vi "Barcode Scanner.vi"(8 "error in":errorcluster, 10 "DUT":string) -> (0 "error in (out)":errorcluster)   [LabVIEW 2024, in "Barcode_Scanner.lvlib"]
doc: "This template is for the Queued Message Handler design pattern.\n\nThe Event Handling Loop generates messages based on user interface actions.\n\nThe Message Handling Loop processes messages generated by the Event Handling Loop, or by other messages. The messages are string values, so new messages can be added easily to the Message Cases case structure in the Message Handling Loop. Each message cluster can also provide an optional value for Message Data, which is a variant that can be converted to whatever message-specific data is required."
uses:
  Barcode_Scanner.lvlib
  controls/Barcode UI Data.ctl
  <vilib>/Instr/_visa.llb/VISA Flush IO Buffer Mask.ctl
  PrivateControls/FGV_Queue_Control.ctl
  Launcher/SubVI/Global 1.vi
  <vilib>/Instr/_visa.llb/VISA Configure Serial Port (Instr).vi
  <vilib>/Utility/error.llb/Error Cluster From Error Code.vi
  <vilib>/regexp/Match Regular Expression.xnode
  <vilib>/ErrorRing/Error Ring.xnode
  support/Message Queue/Barcode Message Queue.lvlib
  support/User Event - Stop/Barcode User Event - Stop.lvlib
  Launcher/Launcher_DTU.lvlib
panel:
  out "read buffer 2":string
  out "Timer 2":i32
  out "Barcode 2":string
  out "status 2":bool
  out "read buffer":string
  in  "Config":string
  out "status":bool
  out "Barcode":string
  out "Timer":i32
  in  "PLC_name":refnum<visa-resource-name>
  out "queue name 2":string
  out "queue name":string
  out "Display <Replace Me>":string
  in  "DigitalWrite":bool
  in  "Digital Read":bool
  in  "Exit":bool
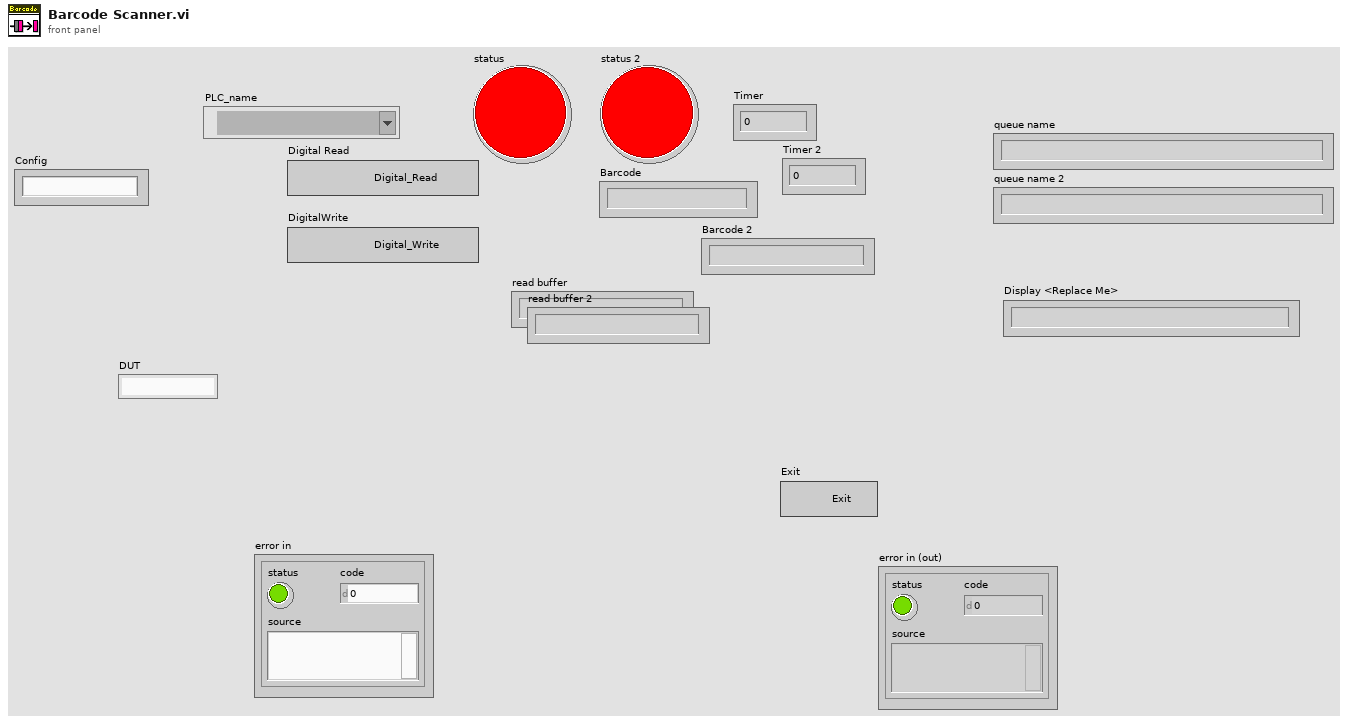
[diagram p1: front panel]
types:
  T1 = typedef "Barcode_Scanner.lvlib/Barcode UI Data.ctl" = cluster{"Config_Path":path, "DUT":i32, "notifier out":refnum<notifier>, "Barcode COM":refnum<visa-resource-name>, "Timer":u32, "queue out":refnum<queue>, "Config":string, "Barcode_path":path, "Barcode_init":bool}
  T2 = typedef "Barcode_Scanner.lvlib/FGV_Queue_Control.ctl" = enum16{"Release", "Get", "Set"}
  T3 = typedef "Barcode_Scanner.lvlib/Barcode Message Queue.lvlib/All Message Queues.ctl" = cluster{"UI":refnum<queue>, "QSM":refnum<queue>}
  T4 = enum16{"Read", "Write", "All_sections", "All_values", "Remove key&section"}
  T5 = cluster{"Message":string, "Message Data":variant}
  T6 = typedef "VISA Flush IO Buffer Mask.ctl" = u16
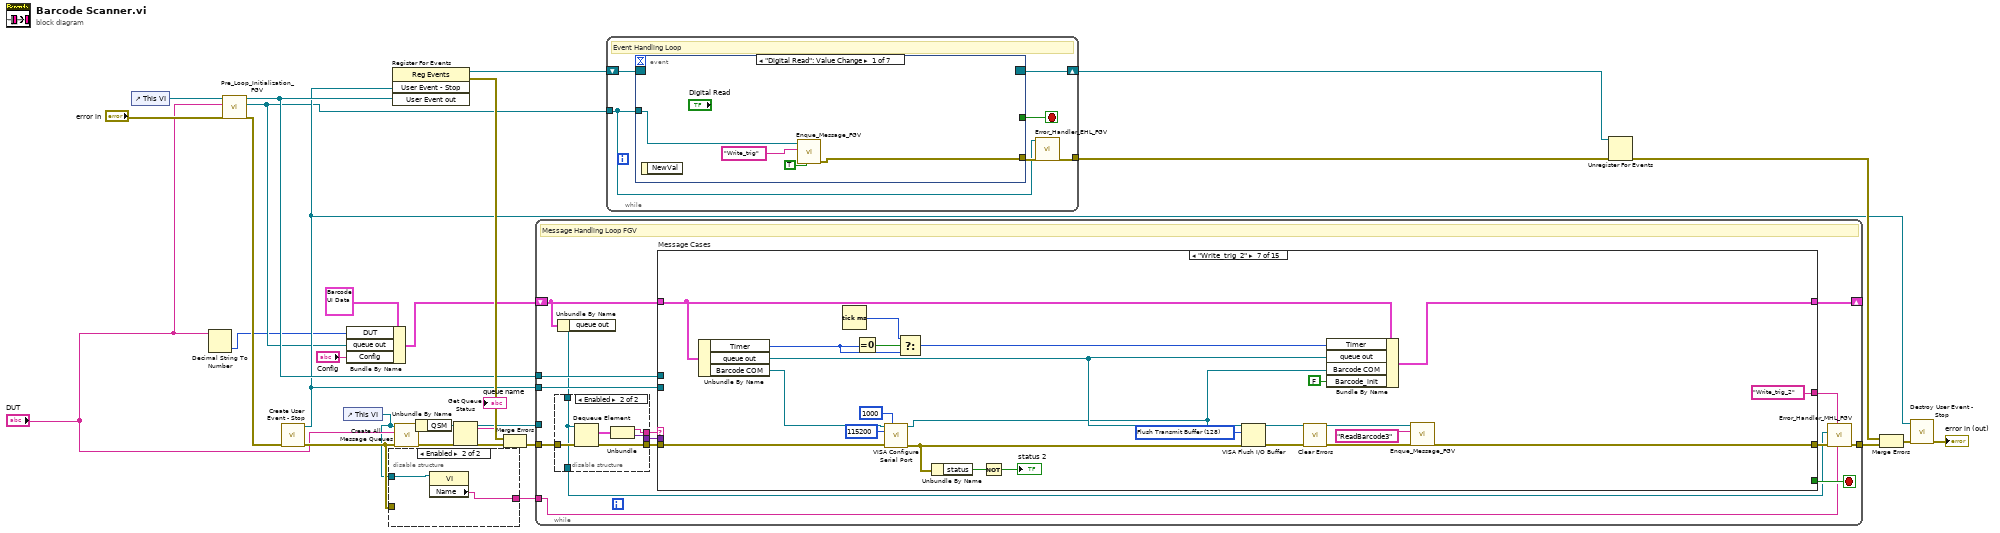
[diagram p0: block diagram]
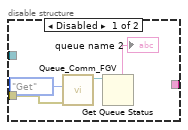
[diagram p2: hidden frame]
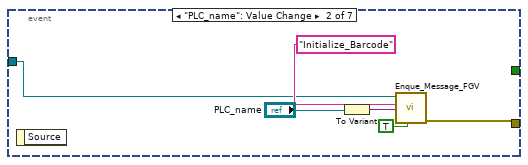
[diagram p3: hidden frame]
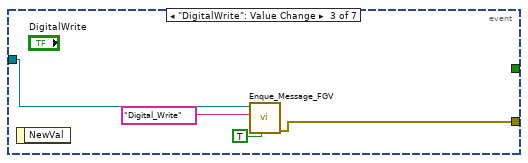
[diagram p4: hidden frame]
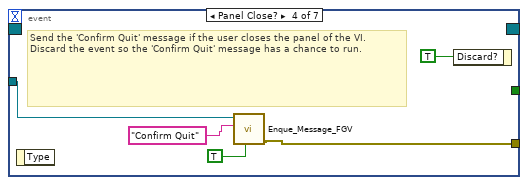
[diagram p5: hidden frame]
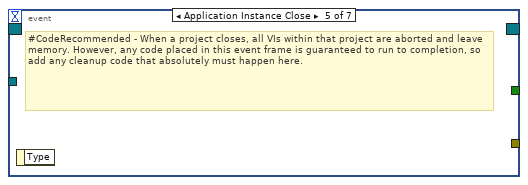
[diagram p6: hidden frame]
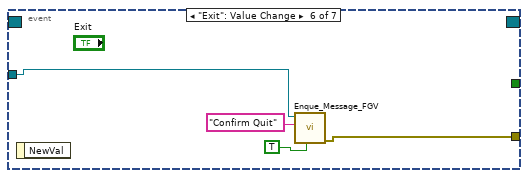
[diagram p7: hidden frame]
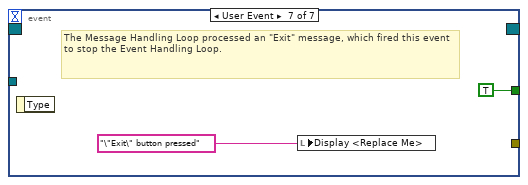
[diagram p8: hidden frame]
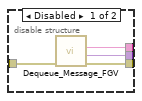
[diagram p9: hidden frame]
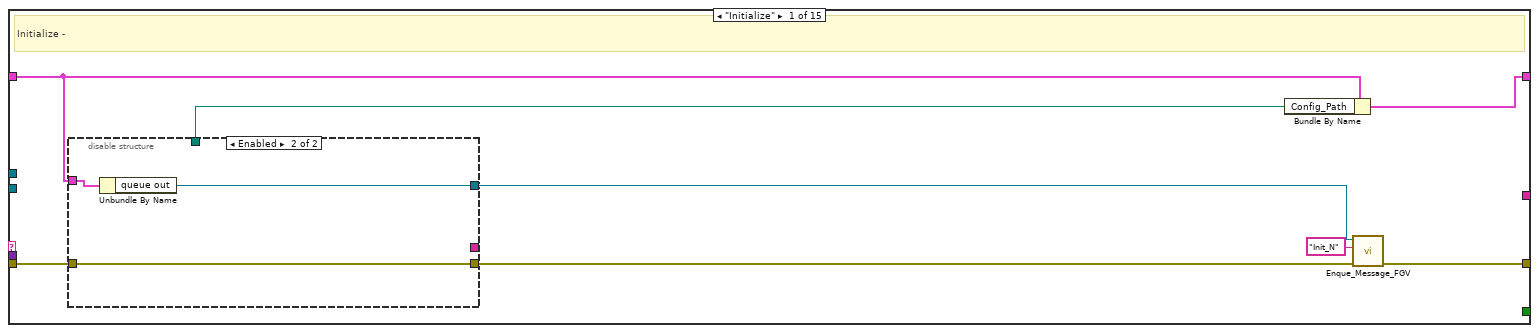
[diagram p10: hidden frame]
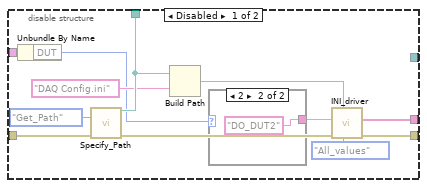
[diagram p11: hidden frame]
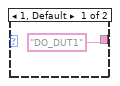
[diagram p12: hidden frame]
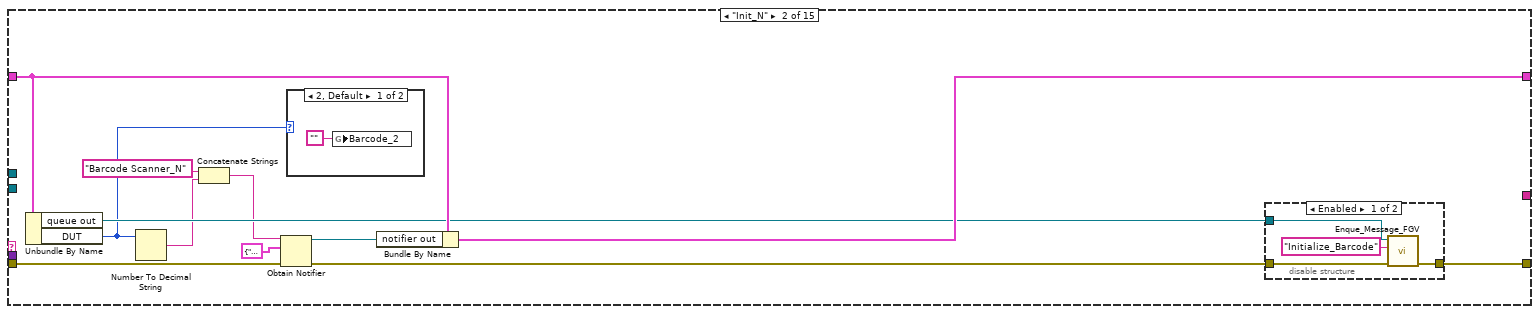
[diagram p13: hidden frame]
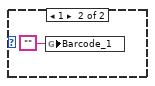
[diagram p14: hidden frame]
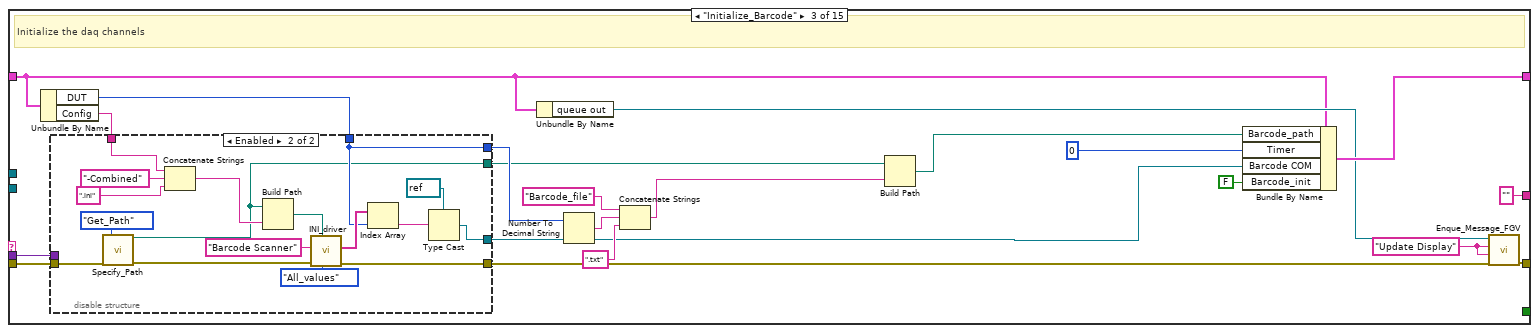
[diagram p16: hidden frame]
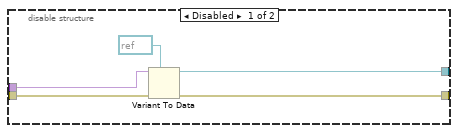
[diagram p17: hidden frame]
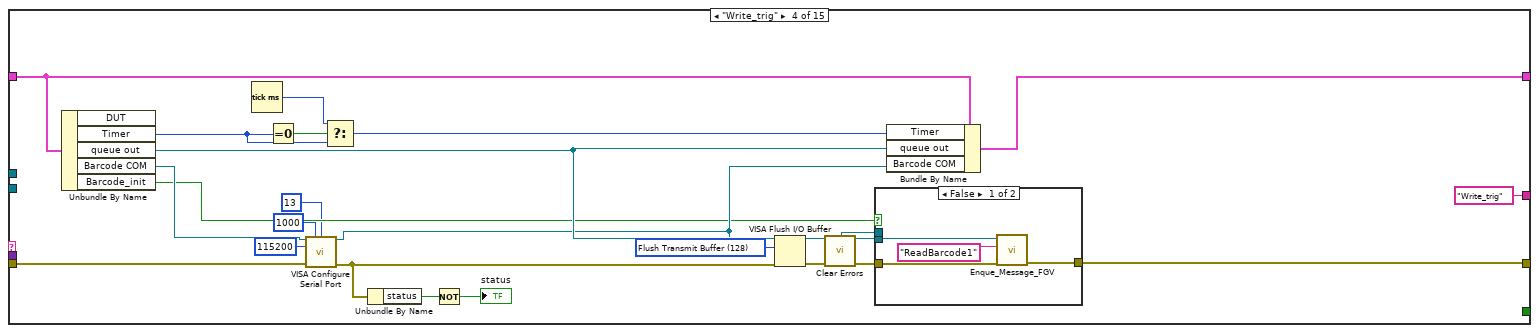
[diagram p18: hidden frame]
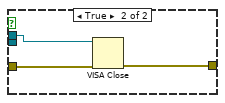
[diagram p19: hidden frame]
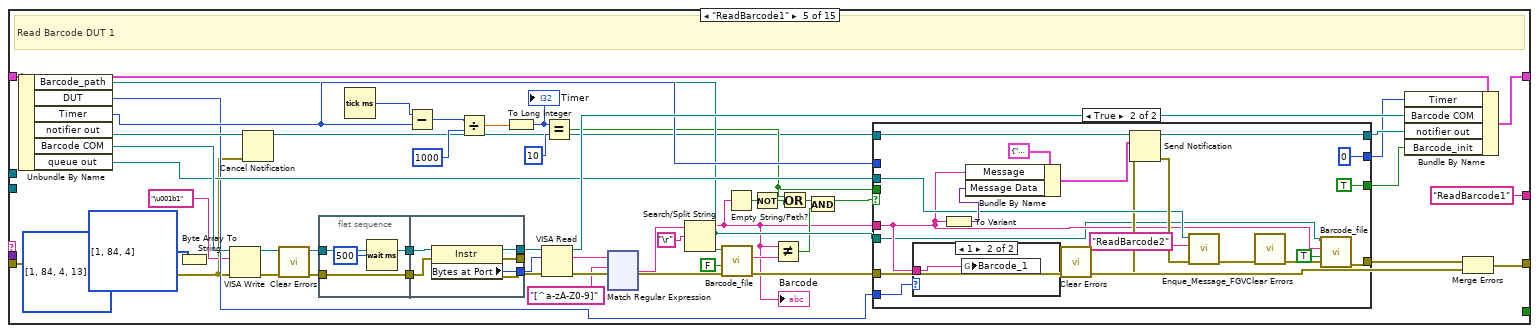
[diagram p20: hidden frame]
diagram:
  n1 = control-ref of="This VI"() -> (w16:refnum<vi>)
  n2 = Decimal String To Number(string="DUT") -> (number=w4:i32)  [unwired: 2 in, 1 out]
  n3 = call "Pre_Loop_Initialization_FGV.vi"("error in (no error)"="error in", "DUT"="DUT", "VI in"=w16) -> ("error out"=w14:errorcluster, "queue out"=w5:refnum<queue>, "User Event out"=w9:refnum<user-event>)  [unwired: 6 in]
  n4 = call "Create User Event - Stop.vi"("error in (no error)"=w14) -> ("error out"=w10:errorcluster, "User Event - Stop"=w8:refnum<user-event>)  [unwired: 9 in]
  n5 = control-ref of="This VI"() -> (w2:refnum<vi>)
  n6 = Bundle By Name(cluster=T1 {"Config_Path"=path "", "DUT"=0, "notifier out"=refnum, "Barcode COM"="", "Timer"=0, "queue out"=refnum, "Config"="", "Barcode_path"=path "", "Barcode_init"=FALSE} ("Data Cluster"), "DUT"=w4, "queue out"=w5, "Config"="Config") -> (w7:T1)
  n7 = disable-structure shown="Enabled" {
    disable-tunnel: w10 -> [w32 _]
    disable-tunnel: w2 -> [_ w34]
    disable-tunnel: [_ w33] -> w1
    frame Disabled {
      n8 = call "Queue_Comm_FGV.vi"("error in (no error)"=w32, "Enum"=FGV_Queue_Control."Get") -> ("queue Out"=w30:refnum<queue>)  [unwired: 8 in, 1 out]
      n9 = Get Queue Status(queue=w30) -> (queue name=→"queue name 2":string)  [unwired: 2 in, 7 out]
    }
    frame Enabled {
      n10 = property class="VI"(reference=w34) -> ("Name"=w33:string)  [unwired: 1 in, 2 out]
    }
  }
  n11 = register-events(w8, w9) -> (reference out=w19:refnum<event-registration>, error out=w17:errorcluster)  [unwired: 2 in]
  n12 = call "Create All Message Queues.vi"("error in (no error)"=w10, "DUT"="DUT", "This VI"=w2) -> ("error out"=w28:errorcluster, "Message Queues out"=w27:T3)  [unwired: 7 in]
  n13 = Unbundle By Name(w27) -> ("QSM"=w25:refnum<queue>)
  n14 = Get Queue Status(queue=w25) -> (queue out=w12:refnum<queue>, queue name=→"queue name":string)  [unwired: 2 in, 6 out]
  n15 = Merge Errors(w17, w28) -> (w18:errorcluster)
  n16 = while {
    tunnel: w12 -> [_]
    shift-right: [w49] -> _
    shift-left: w7 -> [w39]
    tunnel: w9 -> [w47]
    tunnel: w18 -> [w46]
    tunnel: [w41] -> w26
    tunnel: w8 -> [w40]
    tunnel: w1 -> [w35]
    stop <- w48 stop-if-true
    # "Message Handling Loop FGV"
    n17 = Unbundle By Name(w39) -> ("queue out"=w38:refnum<queue>)
    n18 = disable-structure shown="Enabled" {
      disable-tunnel: w46 -> [w53 w59]
      disable-tunnel: [w52 w58] -> w45
      disable-tunnel: [w51 w55] -> w44
      disable-tunnel: [w50 w56] -> w43
      disable-tunnel: w38 -> [_ w54]
      disable-tunnel: [_ w54] -> w37
      frame Disabled {
        n19 = call "Dequeue_Message_FGV.vi"("error in (no error)"=w53) -> ("error out"=w52:errorcluster, "Message Data"=w51:variant, "Message"=w50:string)  [unwired: 8 in]
      }
      frame Enabled {
        n20 = Dequeue Element(queue=w54, error in (no error)=w59) -> (element=w57:T5, error out=w58:errorcluster)  [unwired: 1 in, 2 out]
        n21 = Unbundle(w57) -> ("Message"=w56:string, "Message Data"=w55:variant)
      }
    }
    n22 = case "Message Cases" shown="\"Write_trig_2\"" w43 {
      selector: w43 -> [_ _ _ _ _ _ _ _ _ _ _ _ _ _ w691]
      tunnel: w45 -> [w66 w96 w122 w157 w177 w397 w416 w461 w634 w650 w657 w667 w672 w681 _]
      tunnel: [w67 w90 w124 w163 w222 w402 w422 w469 w639 w651 w657 w661 w674 w678 w692] -> w42
      tunnel: w39 -> [w61 w95 w117 w169 w224 w401 w429 w471 w638 w652 w656 w666 w669 w682 w693]
      tunnel: [w64 w93 w120 w165 w223 w400 w425 w470 w637 w652 w654 w666 w669 w682 w693] -> w49
      tunnel: [_ _ _ _ _ _ _ _ _ _ _ _ _ TRUE _] -> w48
      tunnel: w44 -> [_ _ w121 _ _ _ _ _ _ w649 _ w665 _ _ _]
      tunnel: w47 -> [_ _ _ _ _ _ _ _ _ _ _ _ _ w688 _]
      tunnel: w40 -> [_ _ _ _ _ _ _ _ _ _ _ _ _ w685 _]
      tunnel: [_ _ "" "Write_trig" "ReadBarcode1" "ReadBarcode2" "Write_trig_2" "ReadBarcode3" "ReadBarcode4" "" _ _ _ _ _] -> w36
      frame "Initialize" {
        # "Initialize -"
        n23 = disable-structure shown="Enabled" {
          disable-tunnel: w66 -> [w79 w84]
          disable-tunnel: [w76 w84] -> w63
          disable-tunnel: [w75 _] -> w62
          disable-tunnel: w61 -> [w71 w83]
          disable-tunnel: [w69 _] -> _
          disable-tunnel: [_ w82] -> w60
          frame Disabled {
            n24 = Unbundle By Name(w71) -> ("DUT"=w68:i32)
            n25 = call "Specify_Path.vi"("Path_Enum"=enum16{"Find_Path", "Get_Path"}."Get_Path", "error in (no error)"=w79) -> ("Configurations"=w75:path, "error out"=w78:errorcluster)  [unwired: 6 in, 6 out]
            n26 = Build Path(base path=w75, name or relative path="DAQ Config.ini") -> (appended path=w73:path)
            n27 = case shown="2" w68 {
              tunnel: ["DO_DUT1" ("String") "DO_DUT2" ("String")] -> w70
              frame 1, Default {
              }
              frame 2 {
              }
            }
            n28 = call "INI_driver.vi"("Enum"=T4."All_values", "instrument file path"=w73, "error in (no error)"=w78, "Section"=w70) -> ("error out"=w76:errorcluster, "Values out"=w69:string[])  [unwired: 4 in, 2 out]
          }
          frame Enabled {
            n29 = Unbundle By Name(w83) -> ("queue out"=w82:refnum<queue>)
          }
        }
        n30 = Bundle By Name(cluster=w61, "Config_Path"=w62) -> (w64:T1)
        n31 = call "Enque_Message_FGV.vi"("error in (no error)"=w63, "Message"="Init_N", "queue Out"=w60) -> ("error out"=w67:errorcluster)  [unwired: 8 in]
      }
      frame "Init_N" {
        n32 = Unbundle By Name(w95) -> ("queue out"=w88:refnum<queue>, "DUT"=w85:i32)
        n33 = Number To Decimal String(number=w85) -> (decimal integer string=w86:string)  [unwired: 1 in]
        n34 = Concatenate Strings("Barcode Scanner_N" ("String"), w86) -> (w87:string)
        n35 = Obtain Notifier(name (unnamed)=w87, notification data type=T5 {"Message"="", "Message Data"=variant} ("notification"), error in (no error)=w96) -> (notifier out=w92:refnum<notifier>, error out=w91:errorcluster)  [unwired: 1 in, 1 out]
        n36 = case shown="2, Default" w85 {
          frame 2, Default {
            n37 = global write "Global 1.vi" "Barcode_2"("") -> ()
          }
          frame 1 {
            n38 = global write "Global 1.vi" "Barcode_1"("") -> ()
          }
        }
        n39 = Bundle By Name(cluster=w95, "notifier out"=w92) -> (w93:T1)
        n40 = disable-structure shown="Enabled" {
          disable-tunnel: w91 -> [w101 w103]
          disable-tunnel: [w100 w103] -> w90
          disable-tunnel: w88 -> [w99 _]
          frame Enabled {
            n41 = call "Enque_Message_FGV.vi"("error in (no error)"=w101, "Message"="Initialize_Barcode", "queue Out"=w99) -> ("error out"=w100:errorcluster)  [unwired: 8 in]
          }
          frame Disabled {
          }
        }
      }
      frame "Initialize_Barcode" {
        w123 = "Update Display" ("Message")
        # "Initialize the daq channels"
        n42 = Unbundle By Name(w117) -> ("DUT"=w115:i32, "Config"=w116:string)
        n43 = disable-structure shown="Enabled" {
          disable-tunnel: w122 -> [w129 w136]
          disable-tunnel: [w128 w135] -> w106
          disable-tunnel: w121 -> [w127 _]
          disable-tunnel: [w125 w134] -> w107
          disable-tunnel: w116 -> [_ w133]
          disable-tunnel: w115 -> [_ w131]
          disable-tunnel: [_ w131] -> w114
          disable-tunnel: [_ w130] -> w109
          frame Disabled {
            n44 = Variant To Data(error in=w129, type=refnum<visa-resource-name> refnum ("PLC_name"), Variant=w127) -> (data=w125:refnum<visa-resource-name>, error out=w128:errorcluster)
          }
          frame Enabled {
            n45 = call "Specify_Path.vi"("Path_Enum"=enum16{"Find_Path", "Get_Path"}."Get_Path", "error in (no error)"=w136) -> ("Configurations"=w130:path, "error out"=w143:errorcluster)  [unwired: 6 in, 6 out]
            n46 = Concatenate Strings(w133, "-Combined", ".ini" ("string")) -> (w137:string)
            n47 = Build Path(base path=w130, name or relative path=w137) -> (appended path=w145:path)
            n48 = call "INI_driver.vi"("Enum"=T4."All_values", "instrument file path"=w145, "error in (no error)"=w143, "Section"="Barcode Scanner") -> ("error out"=w135:errorcluster, "Values out"=w141:string[])  [unwired: 4 in, 2 out]
            n49 = Index Array(array=w141, index=w131) -> (element=w140:string)
            n50 = Type Cast(type=refnum<visa-resource-name> refnum ("VISA resource name"), x=w140) -> (*(type *) &x=w134:refnum<visa-resource-name>)
          }
        }
        n51 = Unbundle By Name(w117) -> ("queue out"=w118:refnum<queue>)
        n52 = Number To Decimal String(number=w114) -> (decimal integer string=w111:string)  [unwired: 1 in]
        n53 = Concatenate Strings("Barcode_file", w111, ".txt" ("string")) -> (w113:string)
        n54 = Build Path(base path=w109, name or relative path=w113) -> (appended path=w108:path)
        n55 = Bundle By Name(cluster=w117, "Barcode_path"=w108, "Timer"=u32 0, "Barcode COM"=w107, "Barcode_init"=FALSE) -> (w120:T1)
        n56 = call "Enque_Message_FGV.vi"("error in (no error)"=w106, "Message Data"=w123, "Message"=w123, "queue Out"=w118) -> ("error out"=w124:errorcluster)  [unwired: 7 in]
      }
      frame "Write_trig" {
        w160 = T6 128 items=["Flush Receive Buffer"=16, "Write Transmit Buffer to Device"=32, "Flush Receive Buffer (No I/O)"=64, "Flush Transmit Buffer"=128] ("Mask")
        n57 = Unbundle By Name(w169) -> ("Timer"=w166:u32, "queue out"=w162:refnum<queue>, "Barcode COM"=w156:refnum<visa-resource-name>, "Barcode_init"=w151:bool)  [unwired: 1 out]
        n58 = Tick Count (ms)() -> (millisecond timer value=w167:u32)
        n59 = Equal To 0?(x=w166) -> (x = 0?=w168:bool)
        n60 = call-poly "VISA Configure Serial Port"("VISA resource name"=w156, "timeout (10sec)"=u32 1000, "termination char\n(0xA = '\\n' = LF)"=u8 13 ("termination char\n(0xA = '\\n' = LF)"), "baud rate (9600)"=u32 115200, "error in (no error)"=w157) -> ("VISA resource name out"=w155:refnum<visa-resource-name>, "error out"=w152:errorcluster)  [unwired: 9 in]
        n61 = Select(t=w167, s=w168, f=w166) -> (s? t:f=w164:u32)
        n62 = Unbundle By Name(w152) -> ("status"=w154:bool)
        n63 = Not(x=w154) -> (.not. x?=→"status":bool)
        n64 = VISA Flush I/O Buffer(VISA resource name=w155, mask (16)=w160, error in (no error)=w152) -> (VISA resource name out=w150:refnum<visa-resource-name>, error out=w161:errorcluster)
        n65 = call <vilib>:"Clear Errors.vi"("error in (no error)"=w161) -> ("error out"=w147:errorcluster)  [unwired: 5 in, 1 out]
        n66 = case shown="False" w151 {
          tunnel: [w172 w175] -> w163
          tunnel: w162 -> [w171 _]
          tunnel: w147 -> [w170 w176]
          tunnel: w150 -> [_ w174]
          frame False {
            n67 = call "Enque_Message_FGV.vi"("error in (no error)"=w170, "Message"="ReadBarcode1", "queue Out"=w171) -> ("error out"=w172:errorcluster)  [unwired: 8 in]
          }
          frame True {
            n68 = VISA Close(VISA resource name=w174, error in (no error)=w176) -> (error out=w175:errorcluster)
          }
        }
        n69 = Bundle By Name(cluster=w169, "Timer"=w164, "queue out"=w162, "Barcode COM"=w155) -> (w165:T1)
      }
      frame "ReadBarcode1" {
        (unwired) u8[] [1, 84, 4, 13] ("unsigned byte array")
        # "Read Barcode DUT 1"
        n70 = Unbundle By Name(w224) -> ("Barcode_path"=w191:path, "DUT"=w194:i32, "Timer"=w197:u32, "notifier out"=w221:refnum<notifier>, "Barcode COM"=w214:refnum<visa-resource-name>, "queue out"=w198:refnum<queue>)
        n71 = Byte Array To String(unsigned byte array=u8[] [1, 84, 4]) -> ()  [unwired: 1 out]
        n72 = VISA Write(VISA resource name=w214, write buffer="\u001b1", error in (no error)=w177) -> (VISA resource name out=w213:refnum<visa-resource-name>, error out=w212:errorcluster)  [unwired: 1 out]
        n73 = Cancel Notification(0:w221, 3:w177) -> (8:w178:refnum<notifier>)  [unwired: 2 out]
        n74 = call <vilib>:"Clear Errors.vi"("error in (no error)"=w212) -> ("error out"=w208:errorcluster)  [unwired: 5 in, 1 out]
        n75 = flat-sequence {
          tunnel: w208 -> [w374]
          tunnel: w213 -> [w375]
          tunnel: [w375] -> w210
          tunnel: [w374] -> w209
          tunnel: [w380] -> w218
          tunnel: [w379] -> w217
          tunnel: [w378] -> w216
          tunnel: w210 -> [w377]
          tunnel: w209 -> [w376]
          frame #0 {
            n76 = Wait (ms)(milliseconds to wait=u32 500) -> ()  [unwired: 1 out]
          }
          frame #1 {
            n77 = property class="Instr"(reference=w377, error in=w376) -> (reference out=w380:refnum<visa-resource-name>, error out=w378:errorcluster, "Bytes at Port"=w379:u32)
          }
        }
        n78 = Tick Count (ms)() -> (millisecond timer value=w204:u32)
        n79 = Subtract(x=w204, y=w197) -> (x-y=w203:u32)
        n80 = Divide(x=w203, y=u32 1000) -> (x/y=w201:dbl)
        n81 = To Long Integer(number=w201) -> (32bit integer=w200:i32)
        "Timer" <- w200
        n82 = VISA Read(VISA resource name=w218, byte count=w217, error in (no error)=w216) -> (VISA resource name out=w215:refnum<visa-resource-name>, read buffer=w182:string, error out=w193:errorcluster)  [unwired: 1 out]
        n83 = Equal?(x=w200, y=10) -> (x = y?=w188:bool)
        n84 = xnode "Match Regular Expression"("input string"=w182, "regular expression"="[^a-zA-Z0-9]") -> ("after match"=w181:string)  [unwired: 4 in, 4 out]
        n85 = Search/Split String(string=w181, search string/char (-)="\r") -> (substring before match=w180:string)  [unwired: 1 in, 2 out]
        "Barcode" <- w180
        n86 = call "Barcode_file.vi"("error in"=w193, "Read/Write(Read(F))"=FALSE, "Barcode_Path"=w191) -> ("error out"=w192:errorcluster, "Read_Barcode"=w186:string)  [unwired: 7 in]
        n87 = Empty String/Path?(string/path=w180) -> (empty?=w207:bool)
        n88 = Not(x=w207) -> (.not. x?=w205:bool)
        n89 = Not Equal?(x=w180, y=w186) -> (x != y?=w189:bool)
        n90 = Or(x=w188, y=w205) -> (x .or. y?=w206:bool)
        n91 = And(x=w206, y=w189) -> (x .and. y?=w190:bool)
        n92 = case shown="True" w190 {
          tunnel: w178 -> [w351 w370]
          tunnel: [w349 w353] -> w220
          tunnel: [w351 w367] -> w219
          tunnel: w192 -> [w350 w358]
          tunnel: w180 -> [_ w356]
          tunnel: w198 -> [w348 w362]
          tunnel: w197 -> [w347 _]
          tunnel: [w347 u32 0 ("Timer")] -> w196
          tunnel: w194 -> [_ w361]
          tunnel: w191 -> [_ w355]
          tunnel: w188 -> [w343 _]
          tunnel: [FALSE ("Barcode_init") TRUE ("Barcode_init")] -> w185
          frame False {
            n93 = Select(t="ReadBarcode2" ("Message"), s=w343, f="Write_trig" ("Message")) -> (s? t:f=w344:string)
            n94 = call "Enque_Message_FGV.vi"("error in (no error)"=w350, "Message"=w344, "queue Out"=w348) -> ("error out"=w349:errorcluster)  [unwired: 8 in]
          }
          frame True {
            n95 = case shown="1" w361 {
              tunnel: w356 -> [w371 w372]
              frame 2, Default {
                n96 = global write "Global 1.vi" "Barcode_2"(w371) -> ()
              }
              frame 1 {
                n97 = global write "Global 1.vi" "Barcode_1"(w372) -> ()
              }
            }
            n98 = To Variant(anything=w356) -> (Variant=w366:variant)
            n99 = Bundle By Name(cluster=T5 {"Message"="", "Message Data"=variant} ("notification"), "Message"=w356, "Message Data"=w366) -> (w368:T5)
            n100 = call <vilib>:"Clear Errors.vi"("error in (no error)"=w358) -> ("error out"=w360:errorcluster)  [unwired: 5 in, 1 out]
            n101 = Send Notification(notification=w368, notifier=w370, error in (no error)=w360) -> (notifier out=w367:refnum<notifier>, error out=w363:errorcluster)
            n102 = call "Enque_Message_FGV.vi"("error in (no error)"=w363, "Message"="ReadBarcode2", "queue Out"=w362) -> ("error out"=w354:errorcluster)  [unwired: 8 in]
            n103 = call <vilib>:"Clear Errors.vi"("error in (no error)"=w354) -> ("error out"=w352:errorcluster)  [unwired: 5 in, 1 out]
            n104 = call "Barcode_file.vi"("error in"=w352, "Read/Write(Read(F))"=TRUE, "Barcode"=w356, "Barcode_Path"=w355) -> ("error out"=w353:errorcluster)  [unwired: 6 in, 1 out]
          }
        }
        n105 = Bundle By Name(cluster=w224, "Timer"=w196, "Barcode COM"=w215, "notifier out"=w219, "Barcode_init"=w185) -> (w223:T1)
        n106 = Merge Errors(w220, w192) -> (w222:errorcluster)
      }
      frame "ReadBarcode2" {
        w390 = T6 128 items=["Flush Receive Buffer"=16, "Write Transmit Buffer to Device"=32, "Flush Receive Buffer (No I/O)"=64, "Flush Transmit Buffer"=128] ("Mask")
        # "Read Barcode DUT 2"
        n107 = Unbundle By Name(w401) -> ("notifier out"=w398:refnum<notifier>, "Barcode COM"=w388:refnum<visa-resource-name>, "queue out"=w385:refnum<queue>)
        n108 = property class="Instr"(reference=w388, error in=w397) -> (reference out=w396:refnum<visa-resource-name>, error out=w394:errorcluster, "Bytes at Port"=w395:u32)
        n109 = VISA Read(VISA resource name=w396, byte count=w395, error in (no error)=w394) -> (VISA resource name out=w392:refnum<visa-resource-name>, read buffer=→"read buffer":string, error out=w393:errorcluster)  [unwired: 1 out]
        n110 = VISA Flush I/O Buffer(VISA resource name=w392, mask (16)=w390, error in (no error)=w393) -> (VISA resource name out=w387:refnum<visa-resource-name>, error out=w389:errorcluster)
        n111 = VISA Close(VISA resource name=w387, error in (no error)=w389) -> (error out=w381:errorcluster)
        n112 = Cancel Notification(0:w398, 3:w381) -> (8:w382:refnum<notifier>)  [unwired: 2 out]
        n113 = Flush Queue(queue=w385, error in (no error)=w381) -> (error out=w386:errorcluster)  [unwired: 2 out]
        n114 = Merge Errors(w386, w386) -> (w399:errorcluster)
        n115 = Bundle By Name(cluster=w401, "Barcode COM"=w387, "notifier out"=w382, "Barcode_init"=FALSE) -> (w400:T1)
        n116 = disable-structure shown="Enabled" {
          disable-tunnel: [w406 w407] -> w402
          disable-tunnel: w399 -> [w403 w407]
          frame Disabled {
            n117 = call "Enque_Message_FGV.vi"("error in (no error)"=w403, "Message Data"="Digital_Write1" ("\"Do Something Else\" button pressed"), "Message"="Data_Read") -> ("error out"=w406:errorcluster)  [unwired: 8 in]
          }
          frame Enabled {
          }
        }
      }
      frame "Write_trig_2" {
        w419 = T6 128 items=["Flush Receive Buffer"=16, "Write Transmit Buffer to Device"=32, "Flush Receive Buffer (No I/O)"=64, "Flush Transmit Buffer"=128] ("Mask")
        n118 = Unbundle By Name(w429) -> ("Timer"=w426:u32, "queue out"=w421:refnum<queue>, "Barcode COM"=w415:refnum<visa-resource-name>)
        n119 = Tick Count (ms)() -> (millisecond timer value=w427:u32)
        n120 = Equal To 0?(x=w426) -> (x = 0?=w428:bool)
        n121 = call-poly "VISA Configure Serial Port"("VISA resource name"=w415, "timeout (10sec)"=u32 1000, "baud rate (9600)"=u32 115200, "error in (no error)"=w416) -> ("VISA resource name out"=w414:refnum<visa-resource-name>, "error out"=w411:errorcluster)  [unwired: 10 in]
        n122 = Select(t=w427, s=w428, f=w426) -> (s? t:f=w424:u32)
        n123 = Unbundle By Name(w411) -> ("status"=w413:bool)
        n124 = Not(x=w413) -> (.not. x?=→"status 2":bool)
        n125 = VISA Flush I/O Buffer(VISA resource name=w414, mask (16)=w419, error in (no error)=w411) -> (error out=w420:errorcluster)  [unwired: 1 out]
        n126 = call <vilib>:"Clear Errors.vi"("error in (no error)"=w420) -> ("error out"=w408:errorcluster)  [unwired: 5 in, 1 out]
        n127 = Bundle By Name(cluster=w429, "Timer"=w424, "queue out"=w421, "Barcode COM"=w414, "Barcode_init"=FALSE) -> (w425:T1)
        n128 = call "Enque_Message_FGV.vi"("error in (no error)"=w408, "Message"="ReadBarcode3", "queue Out"=w421) -> ("error out"=w422:errorcluster)  [unwired: 8 in]
      }
      frame "ReadBarcode3" {
        # "Read Barcode DUT 1"
        n129 = Unbundle By Name(w471) -> ("Barcode_path"=w439:path, "DUT"=w440:i32, "Timer"=w443:u32, "notifier out"=w468:refnum<notifier>, "Barcode COM"=w460:refnum<visa-resource-name>, "queue out"=w444:refnum<queue>)  [unwired: 1 out]
        n130 = Byte Array To String(unsigned byte array=u8[] [1, 84, 4, 13]) -> ()  [unwired: 1 out]
        n131 = VISA Write(VISA resource name=w460, write buffer="\u001b1", error in (no error)=w461) -> (VISA resource name out=w459:refnum<visa-resource-name>, error out=w458:errorcluster)  [unwired: 1 out]
        n132 = Cancel Notification(0:w468) -> (8:w430:refnum<notifier>)  [unwired: 1 in, 2 out]
        n133 = call <vilib>:"Clear Errors.vi"("error in (no error)"=w458) -> ("error out"=w454:errorcluster)  [unwired: 5 in, 1 out]
        n134 = flat-sequence {
          tunnel: w454 -> [w615]
          tunnel: w459 -> [w616]
          tunnel: [w616] -> w456
          tunnel: [w615] -> w455
          tunnel: [w621] -> w465
          tunnel: [w620] -> w464
          tunnel: [w619] -> w463
          tunnel: w456 -> [w618]
          tunnel: w455 -> [w617]
          frame #0 {
            n135 = Wait (ms)(milliseconds to wait=u32 500) -> ()  [unwired: 1 out]
          }
          frame #1 {
            n136 = property class="Instr"(reference=w618, error in=w617) -> (reference out=w621:refnum<visa-resource-name>, error out=w619:errorcluster, "Bytes at Port"=w620:u32)
          }
        }
        n137 = Tick Count (ms)() -> (millisecond timer value=w450:u32)
        n138 = Subtract(x=w450, y=w443) -> (x-y=w449:u32)
        n139 = Divide(x=w449, y=u32 1000) -> (x/y=w447:dbl)
        n140 = To Long Integer(number=w447) -> (32bit integer=w446:i32)
        "Timer 2" <- w446
        n141 = VISA Read(VISA resource name=w465, byte count=w464, error in (no error)=w463) -> (VISA resource name out=w462:refnum<visa-resource-name>, read buffer=w435:string, error out=w437:errorcluster)  [unwired: 1 out]
        n142 = Equal?(x=w446, y=10) -> (x = y?=w438:bool)
        n143 = xnode "Match Regular Expression"("input string"=w435, "regular expression"="[^a-zA-Z0-9]") -> ("after match"=w434:string)  [unwired: 4 in, 4 out]
        n144 = Empty String/Path?(string/path=w434) -> (empty?=w453:bool)
        n145 = Not(x=w453) -> (.not. x?=w451:bool)
        n146 = Search/Split String(string=w434, search string/char (-)="\r") -> (substring before match=w432:string)  [unwired: 1 in, 2 out]
        "Barcode 2" <- w432
        n147 = Or(x=w438, y=w451) -> (x .or. y?=w452:bool)
        n148 = case shown="True" w452 {
          tunnel: w430 -> [w597 w611]
          tunnel: [w595 w603] -> w467
          tunnel: [w597 w608] -> w466
          tunnel: w437 -> [w596 w598]
          tunnel: w432 -> [_ w599]
          tunnel: w444 -> [w594 w602]
          tunnel: w443 -> [w593 _]
          tunnel: [w593 u32 0 ("Timer")] -> w442
          tunnel: w440 -> [_ w601]
          tunnel: w439 -> [_ _]
          tunnel: w438 -> [w589 _]
          frame False {
            n149 = Select(t="ReadBarcode4" ("Message"), s=w589, f="Write_trig_2" ("Message")) -> (s? t:f=w590:string)
            n150 = call "Enque_Message_FGV.vi"("error in (no error)"=w596, "Message"=w590, "queue Out"=w594) -> ("error out"=w595:errorcluster)  [unwired: 8 in]
          }
          frame True {
            n151 = case shown="1" w601 {
              tunnel: w599 -> [w612 w613]
              frame 2, Default {
                n152 = global write "Global 1.vi" "Barcode_2"(w612) -> ()
              }
              frame 1 {
                n153 = global write "Global 1.vi" "Barcode_1"(w613) -> ()
              }
            }
            n154 = To Variant(anything=w599) -> (Variant=w607:variant)
            n155 = Bundle By Name(cluster=T5 {"Message"="", "Message Data"=variant} ("notification"), "Message"=w599, "Message Data"=w607) -> (w609:T5)
            n156 = call <vilib>:"Clear Errors.vi"("error in (no error)"=w598) -> ("error out"=w600:errorcluster)  [unwired: 5 in, 1 out]
            n157 = Send Notification(notification=w609, notifier=w611, error in (no error)=w600) -> (notifier out=w608:refnum<notifier>, error out=w604:errorcluster)
            n158 = call "Enque_Message_FGV.vi"("error in (no error)"=w604, "Message"="ReadBarcode4", "queue Out"=w602) -> ("error out"=w603:errorcluster)  [unwired: 8 in]
          }
        }
        n159 = Bundle By Name(cluster=w471, "Timer"=w442, "Barcode COM"=w462, "notifier out"=w466) -> (w470:T1)
        n160 = Merge Errors(w467, w437) -> (w469:errorcluster)
      }
      frame "ReadBarcode4" {
        w627 = T6 128 items=["Flush Receive Buffer"=16, "Write Transmit Buffer to Device"=32, "Flush Receive Buffer (No I/O)"=64, "Flush Transmit Buffer"=128] ("Mask")
        # "Read Barcode DUT 2"
        n161 = Unbundle By Name(w638) -> ("notifier out"=w635:refnum<notifier>, "Barcode COM"=w625:refnum<visa-resource-name>)
        n162 = property class="Instr"(reference=w625, error in=w634) -> (reference out=w633:refnum<visa-resource-name>, error out=w631:errorcluster, "Bytes at Port"=w632:u32)
        n163 = VISA Read(VISA resource name=w633, byte count=w632, error in (no error)=w631) -> (VISA resource name out=w629:refnum<visa-resource-name>, read buffer=→"read buffer 2":string, error out=w630:errorcluster)  [unwired: 1 out]
        n164 = VISA Flush I/O Buffer(VISA resource name=w629, mask (16)=w627, error in (no error)=w630) -> (VISA resource name out=w623:refnum<visa-resource-name>, error out=w626:errorcluster)
        n165 = VISA Close(VISA resource name=w623, error in (no error)=w626) -> (error out=w624:errorcluster)
        n166 = Merge Errors(w624, w624) -> (w636:errorcluster)
        n167 = Bundle By Name(cluster=w638, "Barcode COM"=w623, "notifier out"=w635) -> (w637:T1)
        n168 = disable-structure shown="Enabled" {
          disable-tunnel: [w643 w644] -> w639
          disable-tunnel: w636 -> [w640 w644]
          frame Disabled {
            n169 = call "Enque_Message_FGV.vi"("error in (no error)"=w640, "Message Data"="Digital_Write1" ("\"Do Something Else\" button pressed"), "Message"="Data_Read") -> ("error out"=w643:errorcluster)  [unwired: 8 in]
          }
          frame Enabled {
          }
        }
      }
      frame "Update Display" {
        # "Update Display - Convert the message data to a string to display in the Data Display indicator."
        n170 = Variant To Data(error in=w650, type="", Variant=w649) -> (data=→"Display <Replace Me>":string, error out=w647:errorcluster)
        n171 = Merge Errors(w647) -> (w651:errorcluster)
      }
      frame "Reset" {
        n172 = Unbundle By Name(w656) -> ("DUT"=w655:i32)
        n173 = case shown="1" w655 {
          frame 2, Default {
            n174 = global write "Global 1.vi" "Barcode_2"("") -> ()
          }
          frame 1 {
            n175 = global write "Global 1.vi" "Barcode_1"("") -> ()
          }
        }
        n176 = Bundle By Name(cluster=w656, "Barcode_init"=FALSE) -> (w654:T1)
      }
      frame "Error" {
        # "Error - Display an error dialog. This message is sent by the \"Error Handler\" VIs at the end of other loops in this application."
        n177 = Variant To Data(error in=w667, type=errorcluster {"status"=FALSE, "code"=0, "source"=""} ("error constant"), Variant=w665) -> (data=w663:errorcluster, error out=w662:errorcluster)
        n178 = call <vilib>:"Simple Error Handler.vi"("error in (no error)"=w663) -> ()  [unwired: 4 in, 5 out]
        n179 = call <vilib>:"Clear Errors.vi"("error in (no error)"=w662) -> ("error out"=w660:errorcluster)  [unwired: 5 in, 1 out]
        n180 = Merge Errors(w660) -> (w661:errorcluster)
      }
      frame "Confirm Quit" {
        # "Confirm Quit - Message that can confirm whether or not the user wants to exit the application."
        n181 = Unbundle By Name(w669) -> ("queue out"=w668:refnum<queue>)
        n182 = call "Enque_Message_FGV.vi"("Priority"=TRUE ("Priority Message? (F)"), "error in (no error)"=w672, "Message"="Exit", "queue Out"=w668) -> ("error out"=w673:errorcluster)  [unwired: 7 in]
        n183 = Merge Errors(w673) -> (w674:errorcluster)
      }
      frame "Exit" {
        # "Exit - Exit the application."
        n184 = Unbundle By Name(w682) -> ("Barcode COM"=w676:refnum<visa-resource-name>, "notifier out"=w679:refnum<notifier>, "queue out"=w675:refnum<queue>)
        n185 = Release Notifier(notifier=w679, error in (no error)=w681) -> (error out=w680:errorcluster)  [unwired: 1 in, 2 out]
        n186 = call "Queue_Comm_FGV.vi"("error in (no error)"=w681, "Enum"=FGV_Queue_Control."Release", "queue in"=w675) -> ("error Out"=w686:errorcluster)  [unwired: 7 in, 1 out]
        n187 = VISA Close(VISA resource name=w676, error in (no error)=w680) -> (error out=w677:errorcluster)
        n188 = call "Fire User Event - Stop.vi"("User Event - Stop"=w685) -> ("error out"=w683:errorcluster)  [unwired: 10 in]
        n189 = call "Fire User Event - Stop.vi"("User Event - Stop"=w688) -> ("error out"=w684:errorcluster)  [unwired: 10 in]
        n190 = Merge Errors(w677, w684, w683, w686) -> (w689:errorcluster)
        n191 = call <vilib>:"Clear Errors.vi"("error in (no error)"=w689) -> ("error out"=w678:errorcluster)  [unwired: 5 in, 1 out]
      }
      frame Default {
        # "'Default' case only runs if there is a message that isn't defined in any of the other cases.  Output a programming error."
        n192 = xnode "Error Ring"("parameter 0"=w691) -> ("error out"=w692:errorcluster)
      }
    }
    n193 = call "Error_Handler_MHL_FGV.vi"("VI_name"=w35, "Case"=w36, "error in (no error)"=w42, "queue Out"=w37) -> ("error Out"=w41:errorcluster)  [unwired: 7 in]
  }
  n194 = while {
    shift-right: [w705] -> w22
    shift-left: w19 -> [w706]
    tunnel: [w702] -> w20
    tunnel: w5 -> [w701]
    stop <- w704 stop-if-true
    # "Event Handling Loop"
    n195 = event shown="[0] \"Digital Read\": Value Change" {
      selector: w706 -> [_ _ _ _ _ _ _]
      dyn-events: [_ _ _ _ _ _ _] -> w705
      timeout: _ -> [_ _ _ _ _ _ _]
      tunnel: [_ _ _ _ _ _ TRUE ("Discard?")] -> w704
      tunnel: [w709 w714 w718 w724 _ w729 _] -> w703
      tunnel: w701 -> [w707 w711 w717 w721 _ w726 _]
      event "Digital Read": Value Change {
        n196 = event-data() -> ()  [unwired: 1 in, 1 out]
        n197 = call "Enque_Message_FGV.vi"("Priority"=TRUE ("Priority Message? (F)"), "Message"="Write_trig", "queue Out"=w707) -> ("error out"=w709:errorcluster)  [unwired: 8 in]
      }
      event "PLC_name": Value Change {
        n198 = event-data() -> ()  [unwired: 1 in, 1 out]
        n199 = To Variant(anything="PLC_name") -> (Variant=w713:variant)
        n200 = call "Enque_Message_FGV.vi"("Priority"=TRUE ("Priority Message? (F)"), "Message Data"=w713, "Message"="Initialize_Barcode", "queue Out"=w711) -> ("error out"=w714:errorcluster)  [unwired: 7 in]
      }
      event "DigitalWrite": Value Change {
        n201 = event-data() -> ()  [unwired: 1 in, 1 out]
        n202 = call "Enque_Message_FGV.vi"("Priority"=TRUE ("Priority Message? (F)"), "Message"="Digital_Write", "queue Out"=w717) -> ("error out"=w718:errorcluster)  [unwired: 8 in]
      }
      event Panel Close? {
        # "Send the 'Confirm Quit' message if the user closes the panel of the VI. Discard the event so the 'Confirm Quit' message has a chance to run."
        n203 = event-data() -> ()  [unwired: 1 in, 1 out]
        n204 = call "Enque_Message_FGV.vi"("Priority"=TRUE ("Priority Message? (F)"), "Message"="Confirm Quit", "queue Out"=w721) -> ("error out"=w724:errorcluster)  [unwired: 8 in]
        n205 = event-data("Discard?"=TRUE) -> ()  [unwired: 1 in, 1 out]
      }
      event Application Instance Close {
        # "#CodeRecommended - When a project closes, all VIs within that project are aborted and leave memory. However, any code placed in this event frame is guaranteed to run to completion, so add any cleanup code that absolutely must happen here."
        n206 = event-data() -> ()  [unwired: 1 in, 1 out]
      }
      event "Exit": Value Change {
        n207 = event-data() -> ()  [unwired: 1 in, 1 out]
        n208 = call "Enque_Message_FGV.vi"("Priority"=TRUE ("Priority Message? (F)"), "Message"="Confirm Quit", "queue Out"=w726) -> ("error out"=w729:errorcluster)  [unwired: 8 in]
      }
      event User Event {
        # "The Message Handling Loop processed an \"Exit\" message, which fired this event to stop the Event Handling Loop."
        n209 = event-data() -> ()  [unwired: 1 in, 1 out]
        n210 = local write "Display <Replace Me>"("\"Exit\" button pressed" ("VI Stopped")) -> ()
      }
    }
    n211 = call "Error_Handler_EHL_FGV.vi"("error in (no error)"=w703, "queue Out"=w701) -> ("error Out"=w702:errorcluster)  [unwired: 9 in]
  }
  n212 = Unregister For Events(event registration refnum=w22, error in=w20) -> (error out=w23:errorcluster)
  n213 = Merge Errors(w23, w26) -> (w24:errorcluster)
  n214 = call "Destroy User Event - Stop.vi"("error in (no error)"=w24, "User Event - Stop"=w8) -> ("error out"=→"error in (out)":errorcluster)  [unwired: 9 in]
